vi "broadcastReg-TestUI.vi"() -> ()   [LabVIEW 2017, in "testcase-Broadcast Registry.lvclass"]
uses:
  testcase-Broadcast Registry.lvclass
  src/user.lib/_NEVSTOP/Communicable State Machine(CSM)/_Support/BroadcastRegistry/BroadcastRegistry-Value.ctl
  src/user.lib/_NEVSTOP/Communicable State Machine(CSM)/AdvanceAPI/CSM - Broadcast Message Type.ctl
  src/user.lib/_NEVSTOP/Communicable State Machine(CSM)/Communicable State Machine.lvlib
  src/user.lib/_NEVSTOP/Communicable State Machine(CSM)/_Shared/CSM Shared.lvlib
panel:
  out "Registry":variant
  out "Response Message Info":T1[](array[typedef])
  in  "Boolean":bool
  in  "scripts":string="status@source >> api@target -><register>\nstatus@source >> api2@target -><register>"
  in  "Target":string="target"
  in  "Source":string="source"
  in  "Status":string="status"
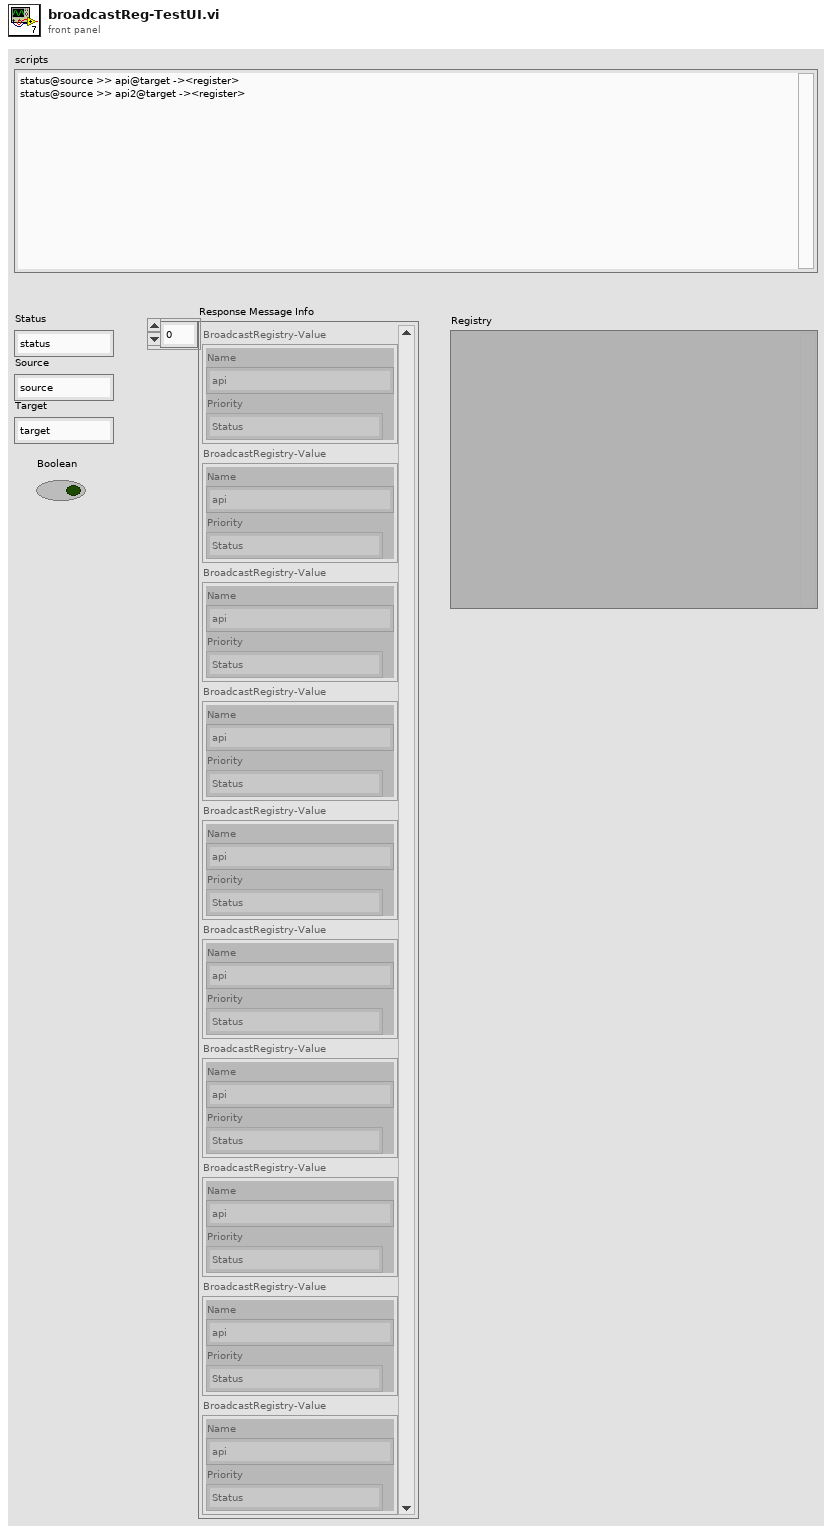
[diagram p1: front panel]
types:
  T1 = typedef "Communicable State Machine.lvlib/BroadcastRegistry-Value.ctl" = cluster{"Name":string, "Priority":T2}
  T2 = typedef "Communicable State Machine.lvlib/CSM - Broadcast Message Type.ctl" = enum16{"Status", "Interrupt"}
  T3 = typedef "Communicable State Machine.lvlib/BroadcastRegistry.ctl" = cluster{"RegistryTable":variant}
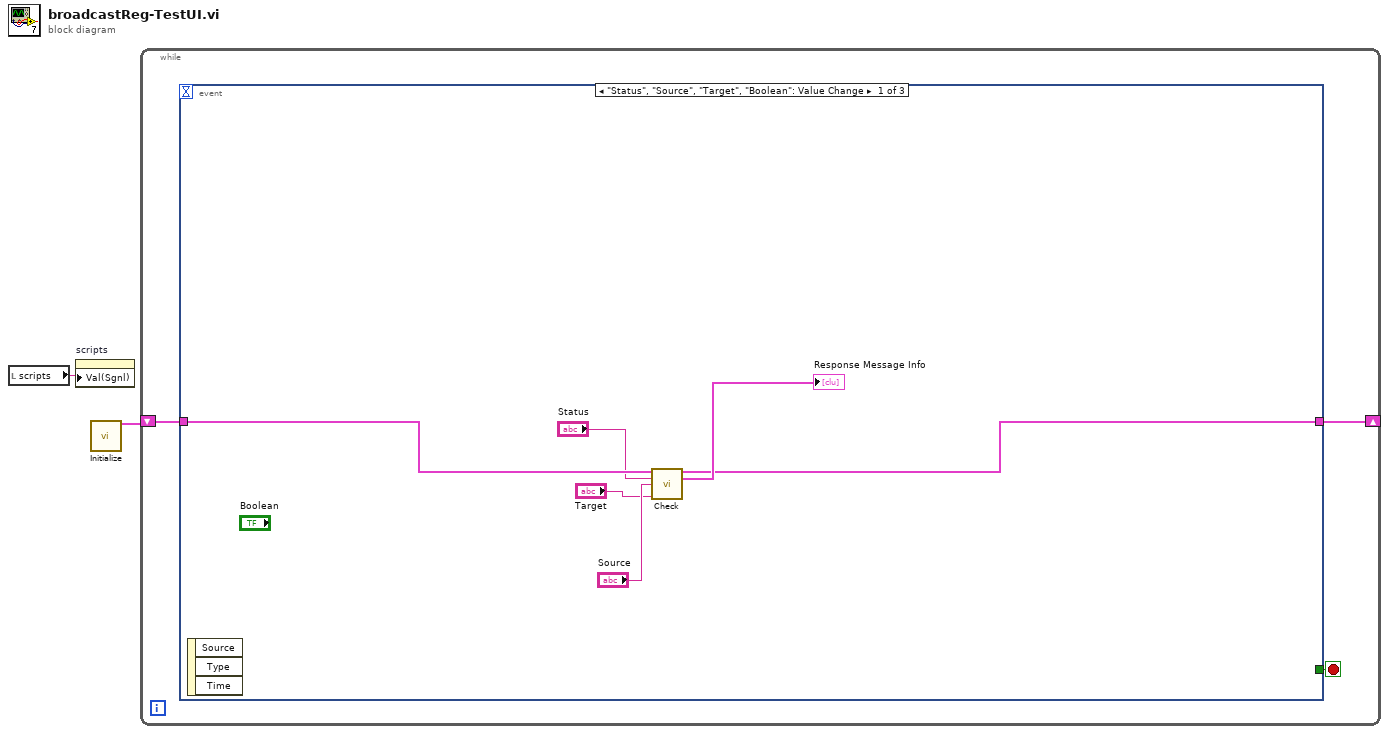
[diagram p0: block diagram]
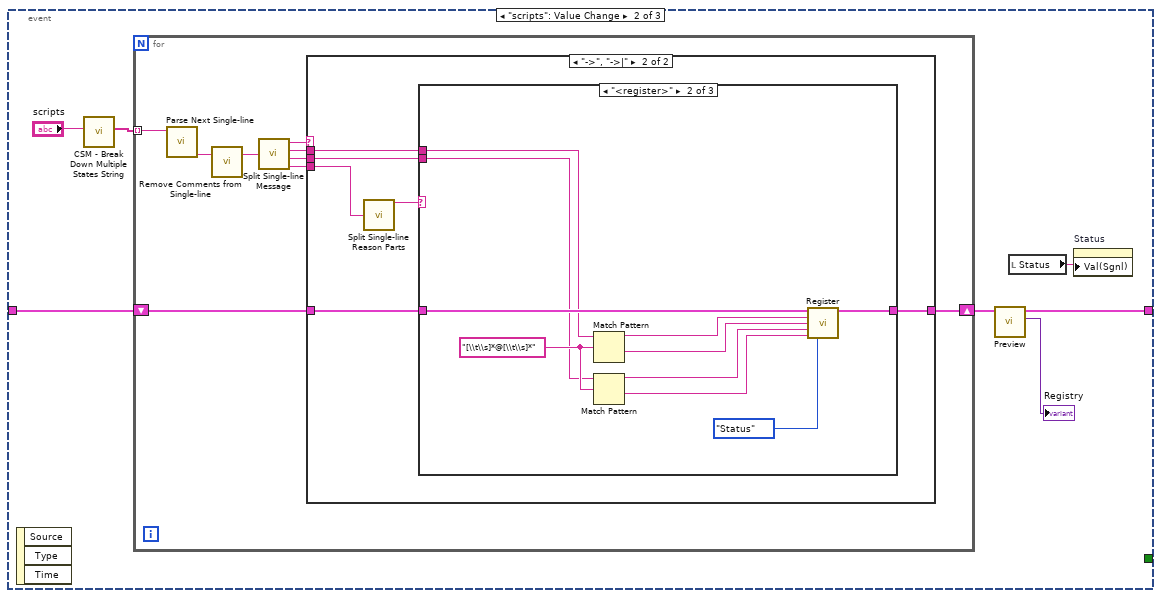
[diagram p2: hidden frame]
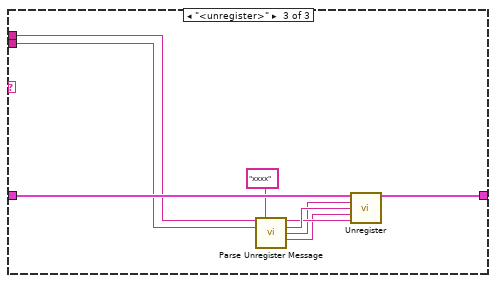
[diagram p5: hidden frame]
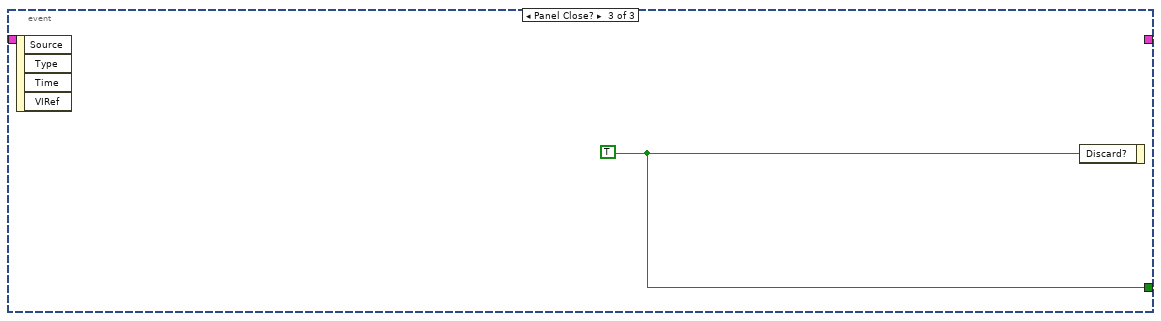
[diagram p6: hidden frame]
diagram:
  n1 = local read "scripts"() -> (w1:string)
  n2 = property on="scripts" class="Str"("Val(Sgnl)"=w1) -> ()  [unwired: 2 in, 2 out]
  n3 = call "Initialize.vi"() -> ("BroadcastRegistry Out"=w2:T3)  [unwired: 15 in]
  n4 = while {
    shift-right: [w3] -> _
    shift-left: w2 -> [w5]
    stop <- w4 stop-if-true
    n5 = event shown="[0] \"Status\", \"Source\", \"Target\", \"Boolean\": Value Change" {
      selector: _ -> [_ _ _]
      dyn-events: _ -> [_ _ _]
      timeout: _ -> [_ _ _]
      tunnel: w5 -> [w11 w15 _]
      tunnel: [_ _ w55] -> w4
      tunnel: [w6 w14 _] -> w3
      event "Status", "Source", "Target", "Boolean": Value Change {
        n6 = event-data() -> ()  [unwired: 1 in, 3 out]
        n7 = call "Check.vi"("BroadcastRegistry In"=w11, "Broadcast"="Status", "SourceCSM"="Source", "TargetCSM"="Target") -> ("BroadcastRegistry Out"=w6:T3, "Response Message Info"=→"Response Message Info":T1[])  [unwired: 10 in]
      }
      event "scripts": Value Change {
        n8 = event-data() -> ()  [unwired: 1 in, 3 out]
        n9 = call "CSM - Break Down Multiple States String.vi"("States"="scripts") -> ("Multiple States"=w18:string[])  [unwired: 10 in]
        n10 = for {
          tunnel: w18 -> [w25] mode=indexing
          shift-right: [w19] -> w16
          shift-left: w15 -> [w20]
          n11 = call "Parse Next Single-line.vi"("States Queue"=w25) -> ("Next Single-line State"=w26:string)  [unwired: 9 in, 1 out]
          n12 = call "Remove Comments from Single-line.vi"("single-line text"=w26) -> ("single-line text without comments"=w27:string)  [unwired: 2 in]
          n13 = call "Split Single-line Message.vi"("single-line text"=w27) -> ("operator"=w24:string, "state"=w23:string, "args"=w22:string, "source/target"=w21:string)  [unwired: 6 in]
          n14 = case shown="\"->\", \"->|\"" w24 {
            tunnel: w23 -> [_ w34]
            tunnel: w22 -> [_ w33]
            tunnel: w21 -> [_ w30]
            tunnel: w20 -> [w28 w32]
            tunnel: [w28 w31] -> w19
            frame "False", Default {
            }
            frame "->", "->|" {
              n15 = call "Split Single-line Reason Parts.vi"("Single-line -& Reason"=w30) -> ("CSM Name"=w29:string)  [unwired: 12 in, 2 out]
              n16 = case shown="\"<register>\"" w29 {
                tunnel: w34 -> [_ w42 w52]
                tunnel: w33 -> [_ w41 w51]
                tunnel: w32 -> [w35 w45 w54]
                tunnel: [w35 w44 w53] -> w31
                frame "False", Default {
                }
                frame "<register>" {
                  w43 = "[\\t\\s]*@[\\t\\s]*" ("regular expression")
                  n17 = Match Pattern(string=w42, regular expression=w43) -> (before substring=w37:string, after substring=w38:string)  [unwired: 1 in, 2 out]
                  n18 = Match Pattern(string=w41, regular expression=w43) -> (before substring=w39:string, after substring=w40:string)  [unwired: 1 in, 2 out]
                  n19 = call "Register.vi"("BroadcastRegistry In"=w45, "Broadcast"=w37, "SourceCSM"=w38, "Name"=w39, "TargetCSM"=w40, "Priority"=CSM_-_Broadcast_Message_Type."Status") -> ("BroadcastRegistry Out"=w44:T3)  [unwired: 9 in]
                }
                frame "<unregister>" {
                  n20 = call "Parse Unregister Message.vi"("State"=w52, "Module Name"="xxxx", "Args"=w51) -> ("Target"=w48:string, "Source"=w49:string, "Status"=w46:string, "Api"=w47:string)  [unwired: 8 in, 1 out]
                  n21 = call "Unregister.vi"("BroadcastRegistry In"=w54, "Broadcast"=w46, "SourceCSM"=w49, "API"=w47, "TargetCSM"=w48) -> ("BroadcastRegistry Out"=w53:T3)  [unwired: 10 in]
                }
              }
            }
          }
        }
        n22 = call "Preview.vi"("BroadcastRegistry In"=w16) -> ("Registry"=→"Registry":variant, "BroadcastRegistry Out"=w14:T3)  [unwired: 8 in, 1 out]
        n23 = local read "Status"() -> (w12:string)
        n24 = property on="Status" class="Str"("Val(Sgnl)"=w12) -> ()  [unwired: 2 in, 2 out]
      }
      event Panel Close? {
        w55 = TRUE ("Discard?")
        n25 = event-data() -> ()  [unwired: 1 in, 4 out]
        n26 = event-data("Discard?"=w55) -> ()  [unwired: 1 in, 1 out]
      }
    }
  }
